vi "Difracción.vi"() -> ()   [LabVIEW 2024]
uses:
  <instrlib>/Arduino UNO/Arduino UNO.lvlib
panel:
  out "XY Graph":cluster{"Y":dbl[], "Y":dbl[]}[](graph)
  out "Intensidad":string
  in  "stop":bool
  in  "VISA resource name":refnum<visa-resource-name>
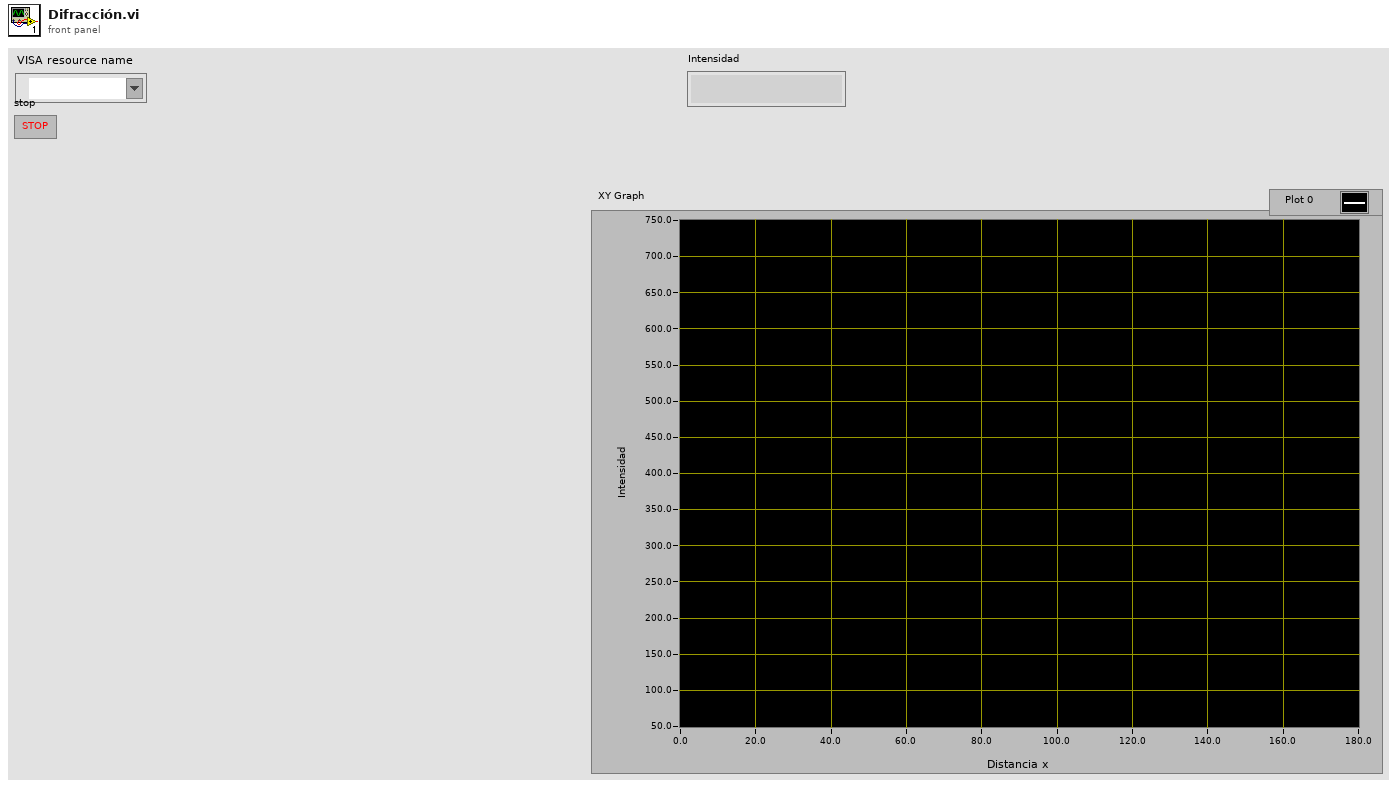
[diagram p1: front panel]
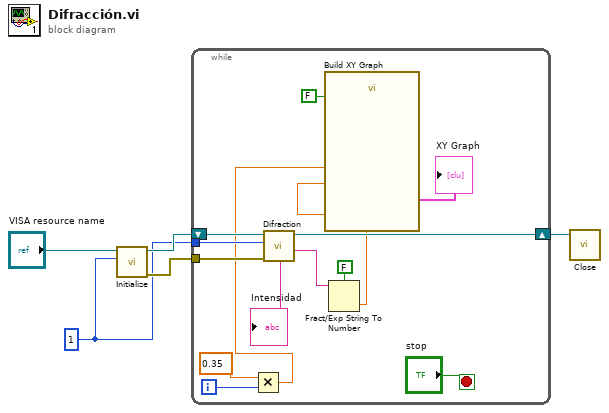
[diagram p0: block diagram]
diagram:
  w2 = u8 1 ("Address")
  n1 = call <instrlib>:"Initialize.vi"("Address"=w2, "VISA resource name"="VISA resource name") -> ("error IO"=w3:errorcluster, "VISA resource name out"=w5:refnum<visa-resource-name>)  [unwired: 7 in, 1 out]
  n2 = while {
    tunnel: w3 -> [w16]
    tunnel: w2 -> [w15]
    shift-right: [w17] -> w4
    shift-left: w5 -> [w18]
    i -> [w11]
    stop <- "stop" stop-if-true
    n3 = Multiply(x=0.35, y=w11) -> (x*y=w10:dbl)
    n4 = call <instrlib>:"Difraction.vi"("error in (no error)"=w16, "Address"=w15, "VISA resource name"=w18) -> ("Intensidad"=w9:string, "VISA resource name out"=w17:refnum<visa-resource-name>)  [unwired: 6 in, 1 out]
    "Intensidad" <- w9
    n5 = Fract/Exp String To Number(use system decimal point (T)=FALSE, string=w9) -> (number=w7:dbl)  [unwired: 2 in, 1 out]
    n6 = call "Build XY Graph"("Reset"=FALSE, "Y Input"=w7, "X Input"=w10) -> ("XY Graph"=→"XY Graph":cluster{"X":dbl[], "Y":dbl[]}[])  [unwired: 7 in, 1 out]
  }
  n7 = call <instrlib>:"Close.vi"("VISA resource name"=w4) -> ()  [unwired: 10 in, 1 out]
